vi "GOOP_ApplyOverlayIcon.vi"(8 "error in (no error)":errorcluster, 10 "IconName(NoPngExtension)":string, 11 "Object":u64) -> (0 "error out":errorcluster)   [LabVIEW 2016]
uses:
  <resource>/Framework/Providers/API/mxLvOverlayState.ctl
  <resource>/Framework/Providers/API/mxLvOverlayAlias.ctl
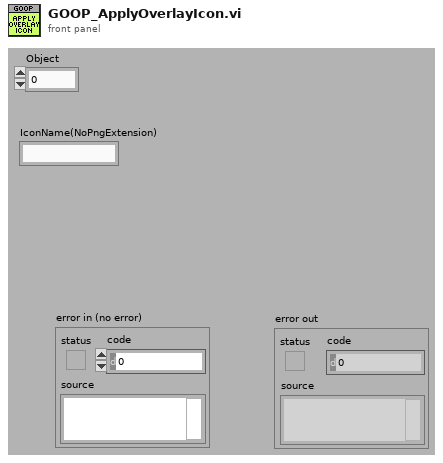
[diagram p1: front panel]
types:
  T1 = typedef "mxLvOverlayAlias.ctl" = cluster{"Overlay Alias":string, "Icon File Name":path}
  T2 = typedef "mxLvOverlayState.ctl" = cluster{"Overlay Alias":string, "Active":bool}
  T3 = typedef "ItemRef.ctl" = u64
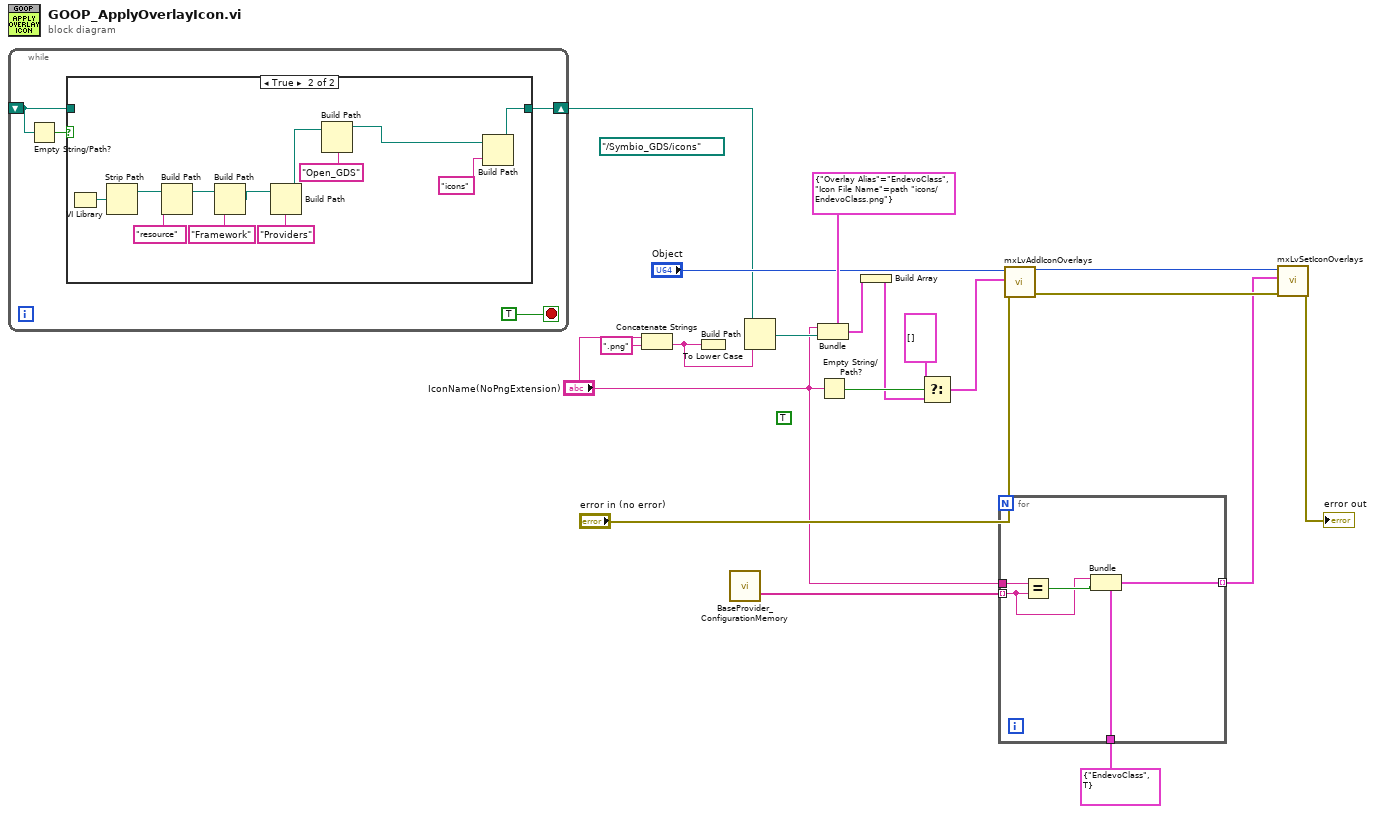
[diagram p0: block diagram]
diagram:
  (unwired) TRUE ("Active")
  (unwired) path "../Symbio_GDS/icons" ("base path")
  n1 = while {
    shift-right: [w22] -> w7
    shift-left: _ -> [w21]
    stop <- TRUE stop-if-true
    n2 = Empty String/Path?(string/path=w21) -> (empty?=w23:bool)
    n3 = case shown="True" w23 {
      tunnel: [w24 w26] -> w22
      tunnel: w21 -> [w24 _]
      frame False {
      }
      frame True {
        n4 = VI Library() -> (path=w28:path)
        n5 = Strip Path(path=w28) -> (stripped path=w29:path)  [unwired: 1 out]
        n6 = Build Path(base path=w29, name or relative path="resource") -> (appended path=w30:path)
        n7 = Build Path(base path=w30, name or relative path="Framework") -> (appended path=w31:path)
        n8 = Build Path(base path=w31, name or relative path="Providers") -> (appended path=w36:path)
        n9 = Build Path(base path=w36, name or relative path="Open_GDS") -> (appended path=w25:path)
        n10 = Build Path(base path=w25, name or relative path="icons") -> (appended path=w26:path)
      }
    }
  }
  n11 = Concatenate Strings("IconName(NoPngExtension)", ".png" ("string")) -> (w6:string)
  n12 = To Lower Case(string=w6) -> ()  [unwired: 1 out]
  n13 = call <resource>:"BaseProvider_ConfigurationMemory.vi"() -> ("ClassItemIconNames"=w8:string[])  [unwired: 13 in, 6 out]
  n14 = Build Path(base path=w7, name or relative path=w6) -> (appended path=w19:path)
  n15 = Bundle(cluster=T1 {"Overlay Alias"="EndevoClass", "Icon File Name"=path "icons/EndevoClass.png"} ("Icon Overlay Alias"), "Overlay Alias"="IconName(NoPngExtension)", "Icon File Name"=w19) -> (w18:T1)
  n16 = Empty String/Path?(string/path="IconName(NoPngExtension)") -> (empty?=w4:bool)
  n17 = Build Array(w18) -> (w3:T1[])
  n18 = Select(t=T1[] [], s=w4, f=w3) -> (s? t:f=w2:T1[])
  n19 = for {
    tunnel: "IconName(NoPngExtension)" -> [w41]
    tunnel: T2 {"Overlay Alias"="EndevoClass", "Active"=TRUE} ("Icon Overlay State") -> [w39]
    tunnel: [w38] -> w9 mode=indexing
    tunnel: w8 -> [w37] mode=indexing
    n20 = Equal?(x=w41, y=w37) -> (x = y?=w40:bool)
    n21 = Bundle(cluster=w39, "Overlay Alias"=w37, "Active"=w40) -> (w38:T2)
  }
  n22 = call <resource>:"mxLvAddIconOverlays.vi"("error in"="error in (no error)", "Overlay Aliases"=w2, "Item"="Object") -> ("error out"=w15:errorcluster, "Item"=w16:T3)  [unwired: 7 in]
  n23 = call <resource>:"mxLvSetIconOverlays.vi"("error in"=w15, "Overlay States"=w9, "Item"=w16) -> ("error out"=→"error out":errorcluster)  [unwired: 7 in, 1 out]
